vi "Add VI Reference Case.vi"(8 "error in":errorcluster, 11 "CSM-Helper in":refnum<class "CSM-Helper.lvclass">) -> (0 "error out":errorcluster, 3 "CSM-Helper out":refnum<class "CSM-Helper.lvclass">)   [LabVIEW 2017, in "CSM-Helper.lvclass"]
doc: "### Add VI Reference Case.vi\n\n-- <b>Controls</b> --\n- <b>CSM-Helper in</b>: CSMHelper input\n\n-- <b>Indicators</b> --\n- <b>CSM-Helper out</b>: CSMHelper output"
uses:
  CSM-Helper.lvclass
  API/Connect Paired Tunnels.vi
  API/Connect Error Wire If not Connected.vi
  API/Connect StateQ Wire If not Connected.vi
  API/Connect Internal Data Wire If not Connected.vi
  API/Connect EventReg Wire If not Connected.vi
  API/Add State Frame.vi
  API/Undo.vi
  API/Stop Undo.vi
  API/Start Undo.vi
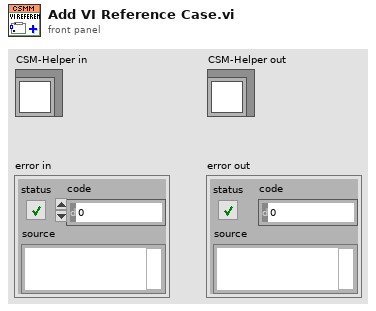
[diagram p1: front panel]
types:
  T1 = enum32{"Invalid", "Standard", "Closed", "Hidden", "Minimized", "Maximized"}
  T2 = enum32{"invalid app kind", "Development System", "Run Time System", "Student Edition", "Embedded LabVIEW", "Evaluation", "Custom"}
  T3 = cluster{"Core":cluster{"Current VI Reference":refnum<vi>, "Close Panel on Exit?":bool, "error":errorcluster}, "Frame":refnum<vi>}
  T4 = cluster{"Current VI Reference":refnum<vi>, "Close Panel on Exit?":bool, "error":errorcluster}
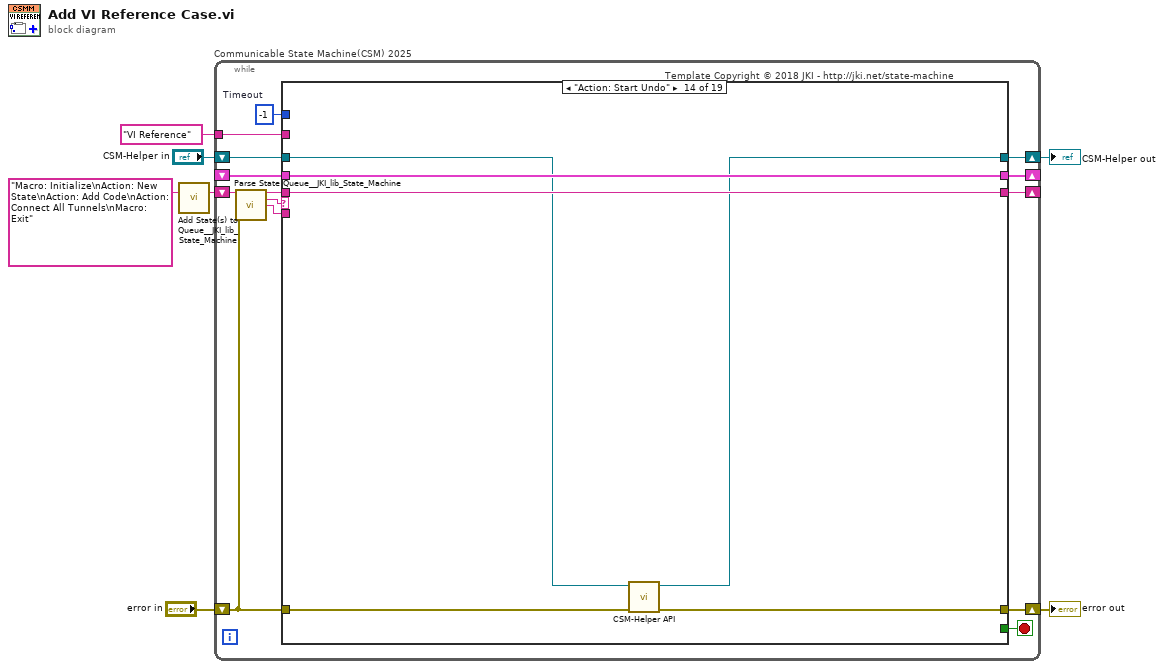
[diagram p0: block diagram]
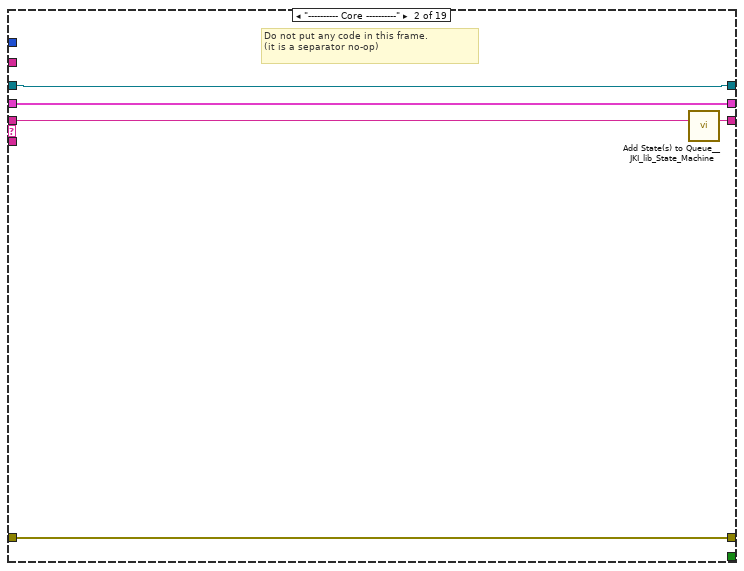
[diagram p3: hidden frame]
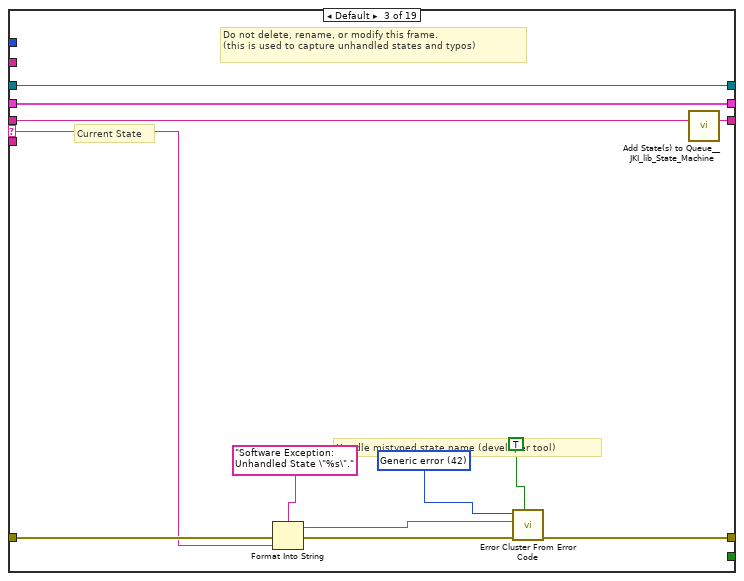
[diagram p4: hidden frame]
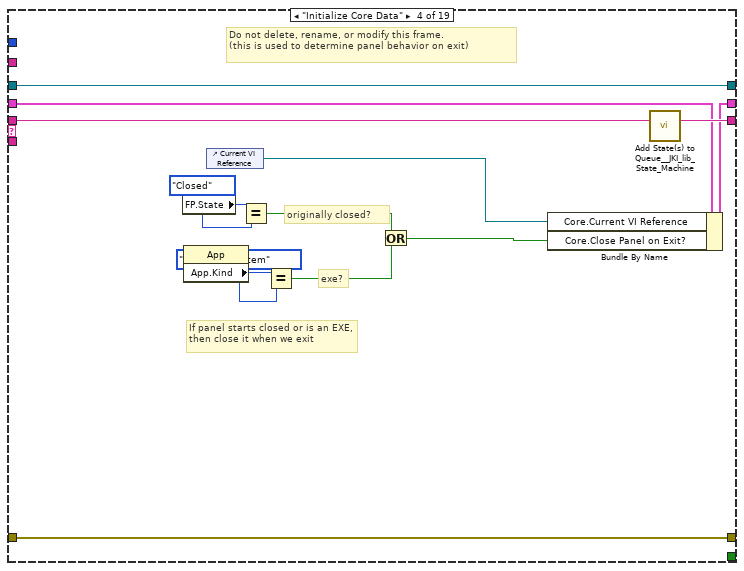
[diagram p5: hidden frame]
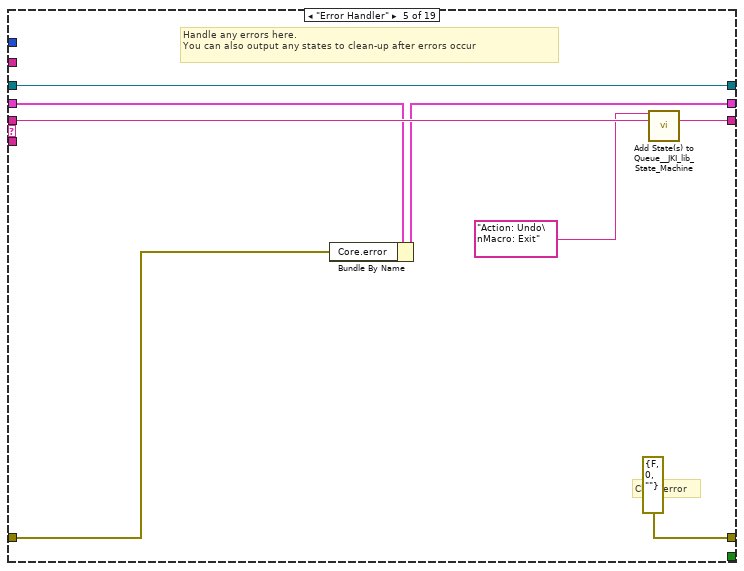
[diagram p6: hidden frame]
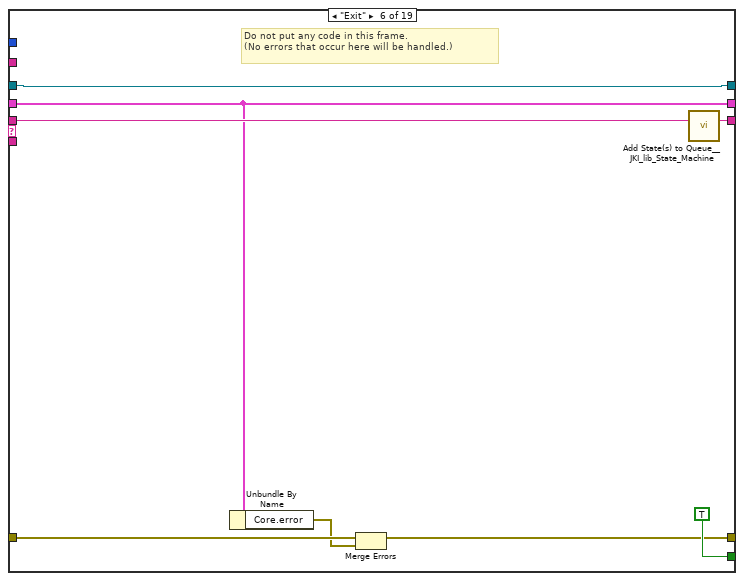
[diagram p7: hidden frame]
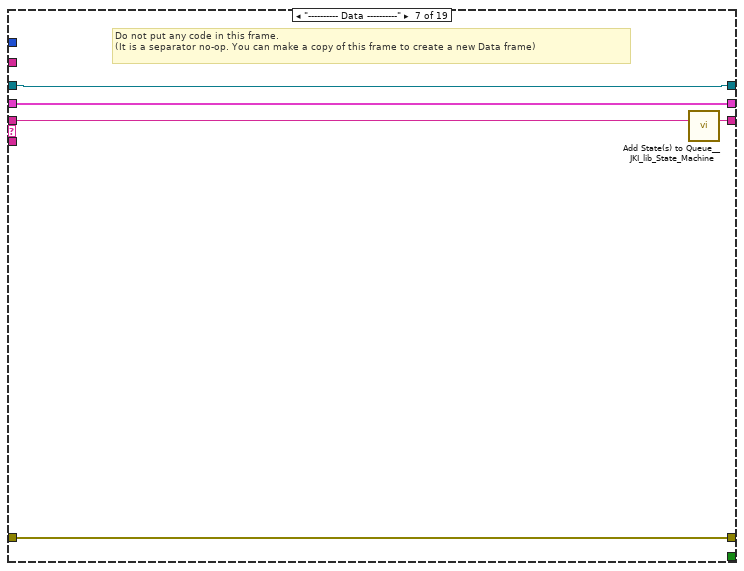
[diagram p8: hidden frame]
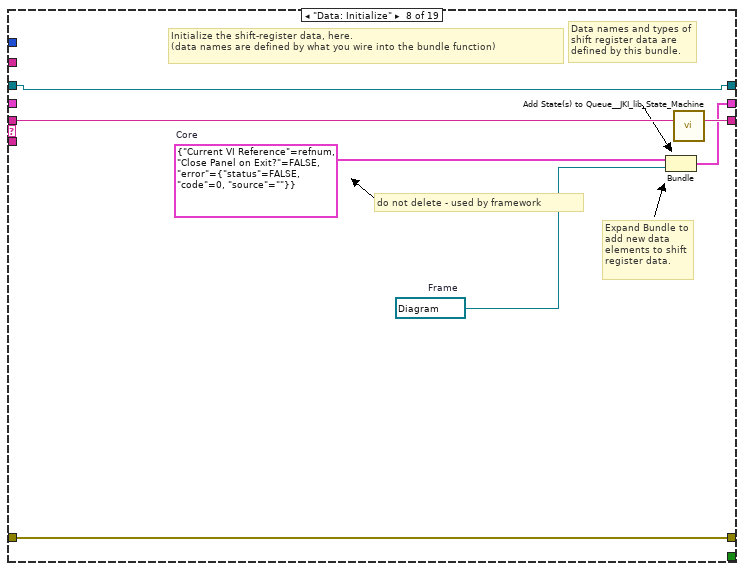
[diagram p9: hidden frame]
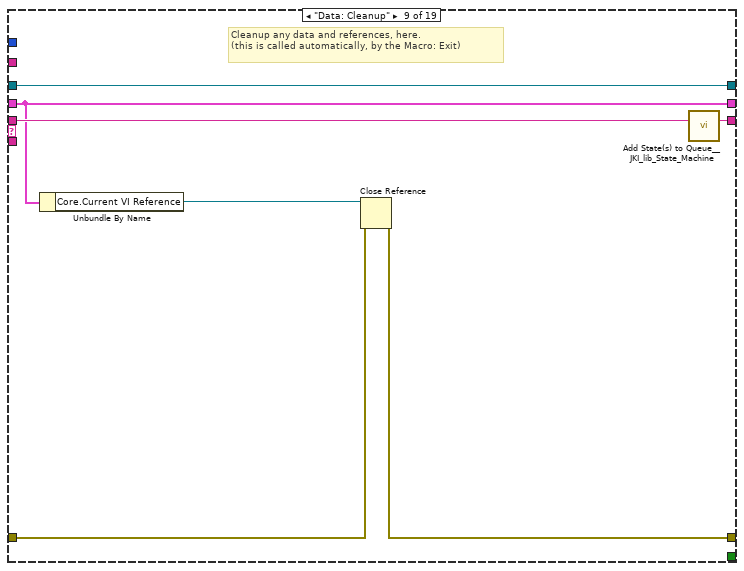
[diagram p10: hidden frame]
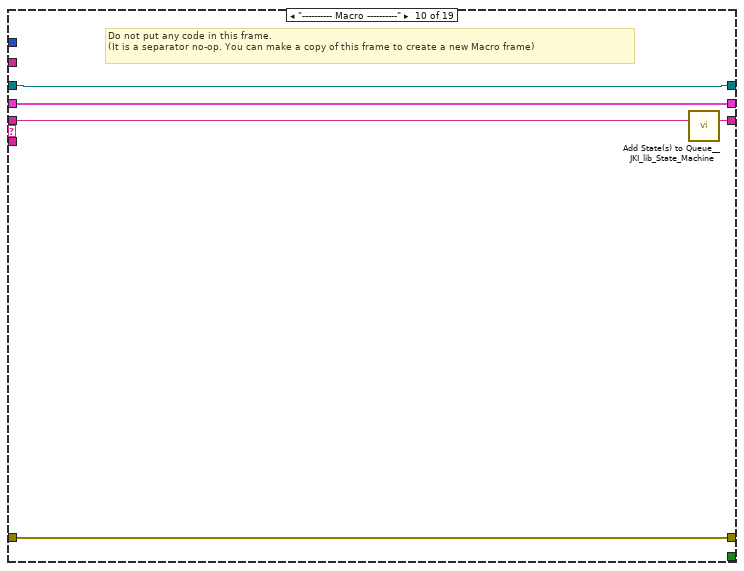
[diagram p11: hidden frame]
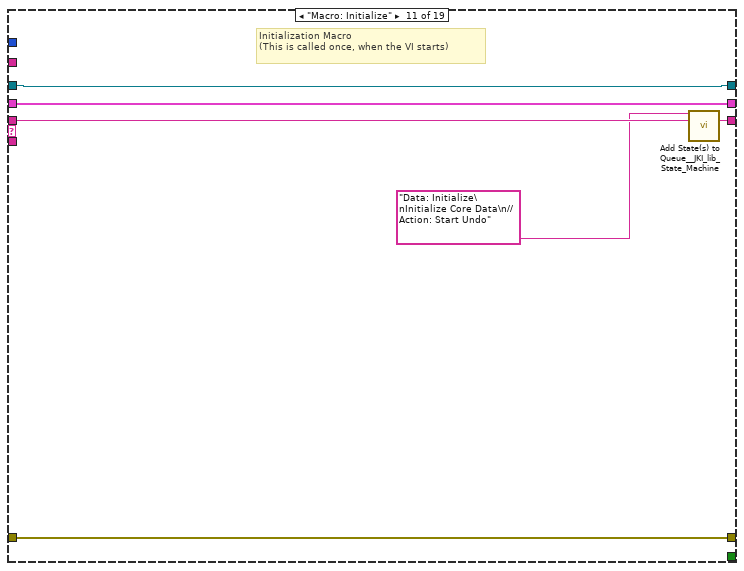
[diagram p12: hidden frame]
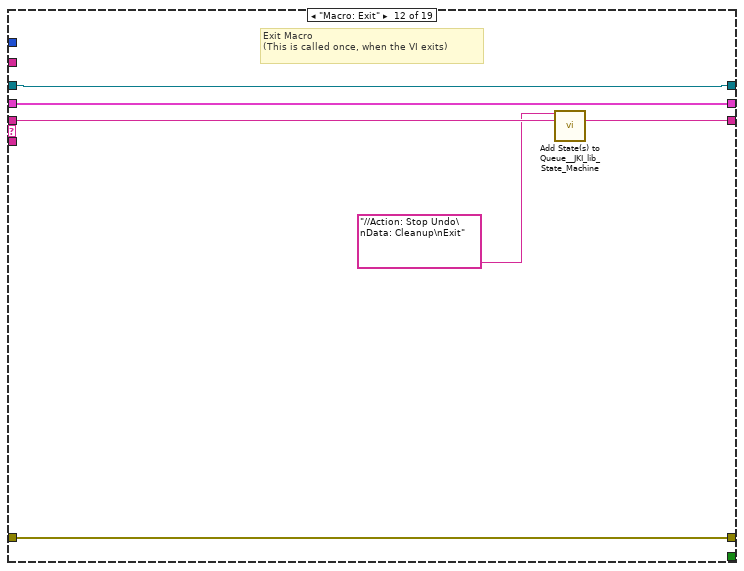
[diagram p13: hidden frame]
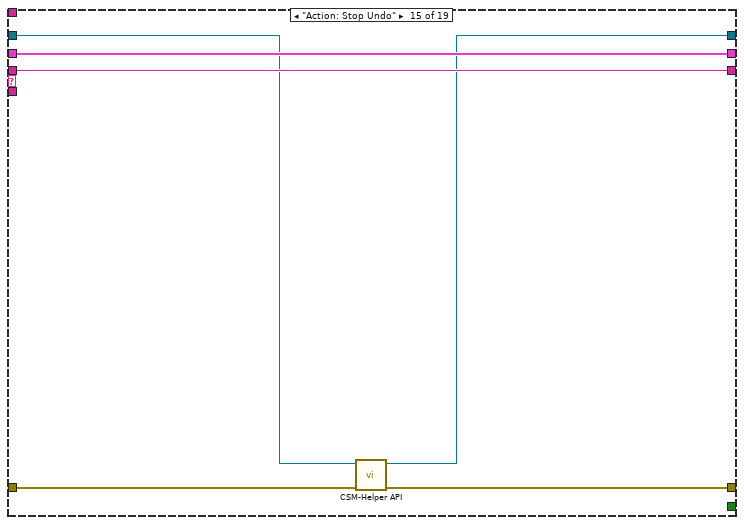
[diagram p15: hidden frame]
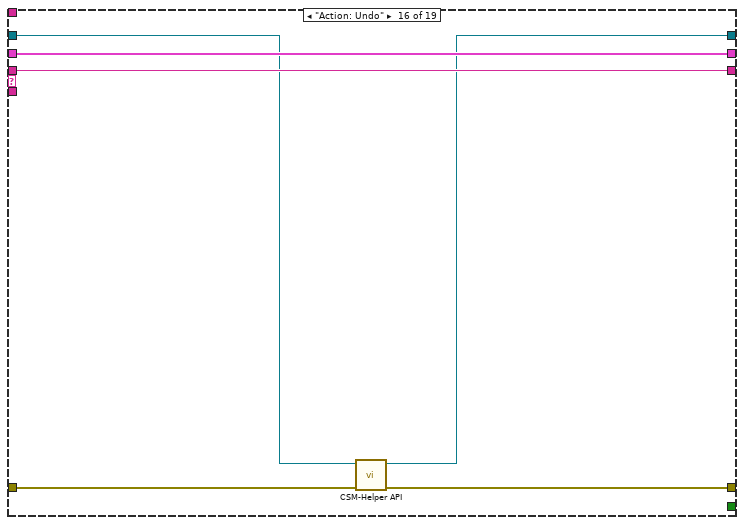
[diagram p16: hidden frame]
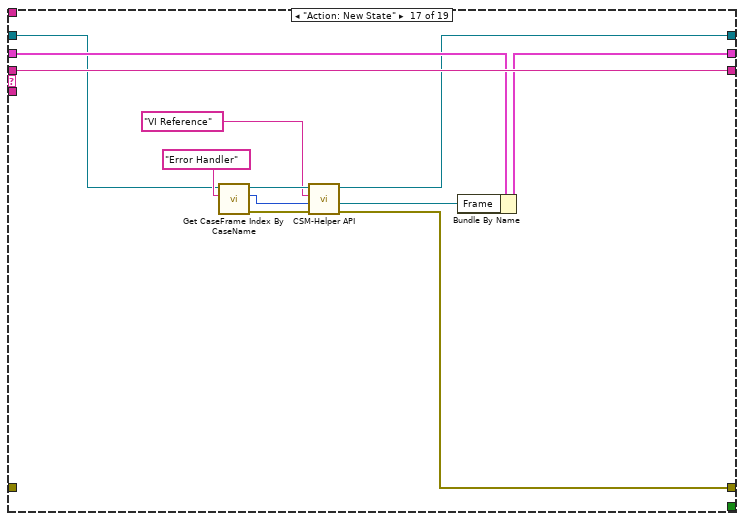
[diagram p17: hidden frame]
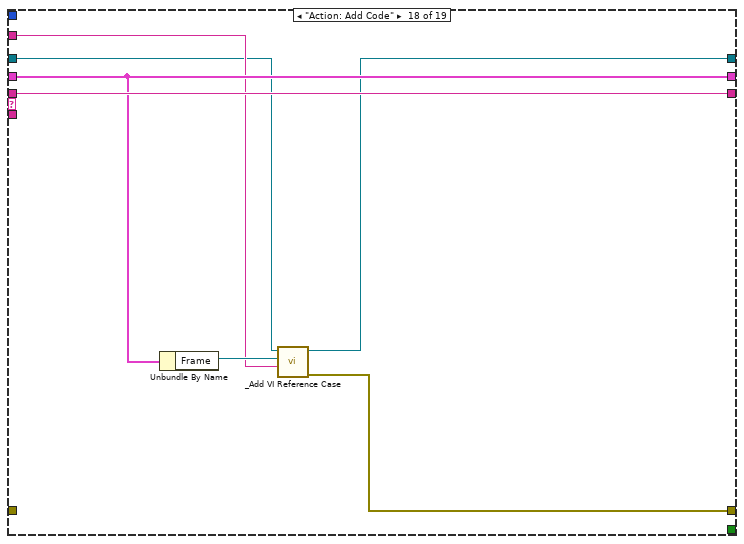
[diagram p18: hidden frame]
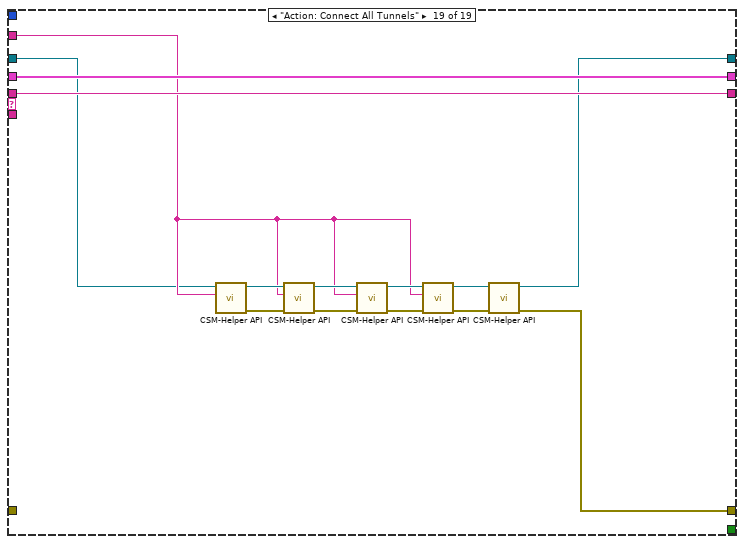
[diagram p19: hidden frame]
diagram:
  n1 = call <vilib>:"Add State(s) to Queue__JKI_lib_State_Machine.vi"("State(s) in (\"\")"="Macro: Initialize\nAction: New State\nAction: Add Code\nAction: Connect All Tunnels\nMacro: Exit") -> ("States Out"=w7:string)  [unwired: 14 in]
  n2 = while "Communicable State Machine(CSM) 2025" {
    shift-right: [w14] -> _
    shift-left: _ -> [w13]
    shift-right: [w17] -> w4
    shift-left: "error in" -> [w11]
    shift-right: [w16] -> _
    shift-left: w7 -> [w18]
    shift-right: [w9] -> w2
    shift-left: "CSM-Helper in" -> [w10]
    tunnel: "VI Reference" ("element") -> [w8]
    stop <- w15 stop-if-true
    w12 = -1  # Timeout
    # "Template Copyright © 2018 JKI - http://jki.net/state-machine"
    n3 = call <vilib>:"Parse State Queue__JKI_lib_State_Machine.vi"("State Queue"=w18, "Error In (no error)"=w11) -> ("Remaining States"=w20:string, "Current State"=w21:string, "Arguments"=w19:string)  [unwired: 11 in]
    n4 = case shown="\"Action: Start Undo\"" w21 {
      selector: w21 -> [_ _ w32 _ _ _ _ _ _ _ _ _ _ _ _ _ _ _ _]
      tunnel: w20 -> [w25 w30 w36 w56 w64 w72 w77 w84 w91 w96 w102 w108 w110 w117 w123 w129 w142 w149 w163]
      tunnel: w19 -> [_ _ _ _ _ _ _ _ _ _ _ _ _ _ _ _ _ _ _]
      tunnel: w13 -> [w23 w27 w34 w49 w61 w66 w74 _ w86 w93 w99 w105 w111 w118 w124 w130 w141 w148 w162]
      tunnel: [w24 w28 w38 w53 errorcluster {"status"=FALSE, "code"=0, "source"=""} ("error out") w67 w75 w81 w87 w94 w100 w106 w109 w115 w121 w127 w135 w143 w153] -> w17
      tunnel: w11 -> [w24 w28 w37 w53 w57 w70 w75 w81 w88 w94 w100 w106 w109 w116 w122 w128 _ _ _]
      tunnel: [w25 w29 w35 w55 w63 w71 w76 w83 w90 w95 w101 w107 w110 w117 w123 w129 w142 w149 w163] -> w16
      tunnel: [_ _ _ _ _ TRUE _ _ _ _ _ _ _ _ _ _ _ _ _] -> w15
      tunnel: [w23 w27 w34 w54 w58 w66 w74 w82 w86 w93 w99 w105 w111 w118 w124 w130 w132 w148 w162] -> w14
      tunnel: w12 -> [_ _ _ _ _ _ _ _ _ _ _ _ _ _ _ _ _ _ _]
      tunnel: w10 -> [w22 w26 w31 w43 w59 w68 w73 w79 w85 w92 w97 w103 w112 w114 w120 w126 w134 w145 w151]
      tunnel: [w22 w26 w31 w43 w59 w68 w73 w79 w85 w92 w97 w103 w112 w113 w119 w125 w133 w144 w150] -> w9
      tunnel: w8 -> [_ _ _ _ _ _ _ _ _ _ _ _ _ _ _ _ _ w146 w152]
      frame "", "Event Structure", "Idle" {
        # "executes when the state queue is empty"
      }
      frame "---------- Core ----------" {
        # "Do not put any code in this frame.\n(it is a separator no-op)"
        n5 = call <vilib>:"Add State(s) to Queue__JKI_lib_State_Machine.vi"("State(s) in (\"\")"=w30) -> ("States Out"=w29:string)  [unwired: 14 in]
      }
      frame Default {
        w41 = 42 items=["No error", "Argument error", "Memory is full", "Out of zone", "End of file", "File already open", "Generic file I/O error", "File not found", "File permission error", "Disk is full", "Duplicate path", "Too many files open", "System feature not enabled", "Resource file not found", "Cannot add resource", "Resource not found", "Image not found", "Image memory error", "Pen does not exist", "Config type invalid", "Config token not found", "Config parse error", "Config memory error", "Bad external code format", "Bad external code offset", "External code not present", "Null window", "Destroy window error", "Null menu", "Print aborted", "Bad print record", "Print driver error", "Windows error during printing", "Memory error during printing", "Print dialog error", "Generic print error", "Invalid device refnum", "Device not found", "Device parameter error", "Device unit error", "Cannot open device", "Device call aborted", "Generic error", "Cancelled by user", "Object ID too low", "Object ID too high", "Object not in heap", "Unknown heap", "Unknown object (invalid DefProc)", "Unknown object (DefProc not in table)", "Message out of range", "Invalid (null) method", "Unknown message", "Manager call not supported", "Bad address", "Network operation in progress", "Network operation timed out", "Connection is busy", "Network attribute not supported", "Network error", "Address in use", "System out of memory", "Connection aborted", "Connection refused", "Not connected", "Already connected", "Connection closed", "Initialization error (interapplication manager)", "Bad occurrence", "Wait on unbound occurrence handler", "Occurrence queue overflow", "Datalog type conflict", "Unused", "Unrecognized type (interapplication manager)", "Memory corrupt", "Failed to make temporary DLL", "Old CIN version", "Drag socket not found", "Failed to load drop-object", "Failed to register OLE object", "Failed to release OLE object", "Format specifier type mismatch", "Unknown format specifier", "Too few format specifiers", "Too many format specifiers", "Scan failed", "Newer CIN version", "Error converting to variant", "Runtime menu error", "Password tampered", "Variant attribute not found", "Incompatible variant data type", "Event data is not available", "Event Store is not present", "Occurrence is not found", "Event Queue is not created", "Event info is not available", "Refnum passed is NULL", "Error retrieving Class GUID", "Error retrieving CoClass GUID", "Error retrieving TypeLib GUID.", "Bad built application magic bytes.", "Specific driver is different from the specific driver associated with the Logical Name.", "There is no session opened to the class driver.", "Max Error", "MAX - Error with config objects", "MAX - Error loading configuration", "MAX - Group not supported"]
        # "Current State"
        # "Do not delete, rename, or modify this frame.\n(this is used to capture unhandled states and typos)"
        # "Handle mistyped state name (developer tool)"
        n6 = Format Into String(format string="Software Exception: Unhandled State \"%s\"." ("message"), error in=w37, w32) -> (resulting string=w40:string, error out=w39:errorcluster)  [unwired: 1 in]
        n7 = call <vilib>:"Error Cluster From Error Code.vi"("show call chain? (False)"=TRUE, "error in (no error)"=w39, "error message (\"\")"=w40, "error code (0)"=w41) -> ("error out"=w38:errorcluster)  [unwired: 5 in]
        n8 = call <vilib>:"Add State(s) to Queue__JKI_lib_State_Machine.vi"("State(s) in (\"\")"=w36) -> ("States Out"=w35:string)  [unwired: 14 in]
      }
      frame "Initialize Core Data" {
        # "Do not delete, rename, or modify this frame.\n(this is used to determine panel behavior on exit)"
        # "originally closed?"
        # "exe?"
        # "If panel starts closed or is an EXE, then close it when we exit"
        n9 = property class="VI"() -> ("FP.State"=w46:T1)  [unwired: 2 in, 2 out]
        n10 = property class="App"() -> ("App.Kind"=w52:T2)  [unwired: 2 in, 2 out]
        n11 = control-ref of="Current VI Reference"() -> (w47:refnum<vi>)
        n12 = Equal?(x=w46, y=T1."Closed" ("Front Panel Window:State")) -> (x = y?=w44:bool)
        n13 = Equal?(x=w52, y=T2."Run Time System" ("Application:Kind")) -> (x = y?=w50:bool)
        n14 = Or(x=w44, y=w50) -> (x .or. y?=w48:bool)
        n15 = Bundle By Name(cluster=w49, "Core.Current VI Reference"=w47, "Core.Close Panel on Exit?"=w48) -> (w54:T3)
        n16 = call <vilib>:"Add State(s) to Queue__JKI_lib_State_Machine.vi"("State(s) in (\"\")"=w56) -> ("States Out"=w55:string)  [unwired: 14 in]
      }
      frame "Error Handler" {
        # "Handle any errors here.\nYou can also output any states to clean-up after errors occur"
        # "Clear error"
        n17 = Bundle By Name(cluster=w61, "Core.error"=w57) -> (w58:T3)
        n18 = call <vilib>:"Add State(s) to Queue__JKI_lib_State_Machine.vi"("State(s) in Front (\"\")"="Action: Undo\nMacro: Exit", "State(s) in (\"\")"=w64) -> ("States Out"=w63:string)  [unwired: 13 in]
      }
      frame "Exit" {
        # "Do not put any code in this frame.\n(No errors that occur here will be handled.)"
        n19 = Unbundle By Name(w66) -> ("Core.error"=w65:errorcluster)
        n20 = Merge Errors(w70, w65) -> (w67:errorcluster)
        n21 = call <vilib>:"Add State(s) to Queue__JKI_lib_State_Machine.vi"("State(s) in (\"\")"=w72) -> ("States Out"=w71:string)  [unwired: 14 in]
      }
      frame "---------- Data ----------" {
        # "Do not put any code in this frame.\n(It is a separator no-op. You can make a copy of this frame to create a new Data frame)"
        n22 = call <vilib>:"Add State(s) to Queue__JKI_lib_State_Machine.vi"("State(s) in (\"\")"=w77) -> ("States Out"=w76:string)  [unwired: 14 in]
      }
      frame "Data: Initialize" {
        w78 = refnum<vi> refnum  # Frame
        w80 = T4 {"Current VI Reference"=refnum, "Close Panel on Exit?"=FALSE, "error"={"status"=FALSE, "code"=0, "source"=""}}  # Core
        # "do not delete - used by framework"
        # "Expand Bundle to add new data elements to shift register data."
        # "Data names and types of shift register data are defined by this bundle."
        # "Initialize the shift-register data, here.\n(data names are defined by what you wire into the bundle function)"
        n23 = Bundle("Core"=w80, "Frame"=w78) -> (w82:T3)  [unwired: 1 in]
        n24 = call <vilib>:"Add State(s) to Queue__JKI_lib_State_Machine.vi"("State(s) in (\"\")"=w84) -> ("States Out"=w83:string)  [unwired: 14 in]
      }
      frame "Data: Cleanup" {
        # "Cleanup any data and references, here.\n(this is called automatically, by the Macro: Exit)"
        n25 = Unbundle By Name(w86) -> ("Core.Current VI Reference"=w89:refnum<vi>)
        n26 = Close Reference(reference=w89, error in (no error)=w88) -> (error out=w87:errorcluster)
        n27 = call <vilib>:"Add State(s) to Queue__JKI_lib_State_Machine.vi"("State(s) in (\"\")"=w91) -> ("States Out"=w90:string)  [unwired: 14 in]
      }
      frame "---------- Macro ----------" {
        # "Do not put any code in this frame.\n(It is a separator no-op. You can make a copy of this frame to create a new Macro frame)"
        n28 = call <vilib>:"Add State(s) to Queue__JKI_lib_State_Machine.vi"("State(s) in (\"\")"=w96) -> ("States Out"=w95:string)  [unwired: 14 in]
      }
      frame "Macro: Initialize" {
        # "Initialization Macro\n(This is called once, when the VI starts)"
        n29 = call <vilib>:"Add State(s) to Queue__JKI_lib_State_Machine.vi"("State(s) in Front (\"\")"="Data: Initialize\nInitialize Core Data\n//Action: Start Undo", "State(s) in (\"\")"=w102) -> ("States Out"=w101:string)  [unwired: 13 in]
      }
      frame "Macro: Exit" {
        # "Exit Macro\n(This is called once, when the VI exits)"
        n30 = call <vilib>:"Add State(s) to Queue__JKI_lib_State_Machine.vi"("State(s) in Front (\"\")"="//Action: Stop Undo\nData: Cleanup\nExit", "State(s) in (\"\")"=w108) -> ("States Out"=w107:string)  [unwired: 13 in]
      }
      frame "--------- Action -----------" {
      }
      frame "Action: Start Undo" {
        n31 = call-poly "CSM-Helper API.vi"("error in (no error)"=w116, "CSM-Helper in"=w114) -> ("error out"=w115:errorcluster, "CSM-Helper out"=w113:refnum<class "CSM-Helper.lvclass">)  [unwired: 8 in]
      }
      frame "Action: Stop Undo" {
        n32 = call-poly "CSM-Helper API.vi"("error in (no error)"=w122, "CSM-Helper in"=w120) -> ("error out"=w121:errorcluster, "CSM-Helper out"=w119:refnum<class "CSM-Helper.lvclass">)  [unwired: 8 in]
      }
      frame "Action: Undo" {
        n33 = call-poly "CSM-Helper API.vi"("error in (no error)"=w128, "CSM-Helper in"=w126) -> ("error out"=w127:errorcluster, "CSM-Helper out"=w125:refnum<class "CSM-Helper.lvclass">)  [unwired: 8 in]
      }
      frame "Action: New State" {
        n34 = call "Get CaseFrame Index By CaseName.vi"("CASE"="Error Handler" ("Frame Name"), "CSM-Helper in"=w134) -> ("error out"=w137:errorcluster, "index"=w140:i32, "CSM-Helper out"=w138:refnum<class "CSM-Helper.lvclass">)  [unwired: 6 in, 1 out]
        n35 = call-poly "CSM-Helper API.vi"("error in (no error)"=w137, "index(-1, use same group)"=w140, "element"="VI Reference", "CSM-Helper in"=w138) -> ("error out"=w135:errorcluster, "Add Frame"=w131:refnum<vi>, "CSM-Helper out"=w133:refnum<class "CSM-Helper.lvclass">)  [unwired: 5 in]
        n36 = Bundle By Name(cluster=w141, "Frame"=w131) -> (w132:T3)
      }
      frame "Action: Add Code" {
        n37 = Unbundle By Name(w148) -> ("Frame"=w147:refnum<vi>)
        n38 = call "_Add VI Reference Case.vi"("element"=w146, "Add Frame"=w147, "CSM-Helper in"=w145) -> ("error out"=w143:errorcluster, "CSM-Helper out"=w144:refnum<class "CSM-Helper.lvclass">)  [unwired: 7 in]
      }
      frame "Action: Connect All Tunnels" {
        n39 = call-poly "CSM-Helper API.vi"("case"=w152, "CSM-Helper in"=w151) -> ("error out"=w159:errorcluster, "CSM-Helper out"=w158:refnum<class "CSM-Helper.lvclass">)  [unwired: 8 in]
        n40 = call-poly "CSM-Helper API.vi"("error in (no error)"=w159, "case"=w152, "CSM-Helper in"=w158) -> ("error out"=w156:errorcluster, "CSM-Helper out"=w157:refnum<class "CSM-Helper.lvclass">)  [unwired: 7 in]
        n41 = call-poly "CSM-Helper API.vi"("error in (no error)"=w156, "case"=w152, "CSM-Helper in"=w157) -> ("error out"=w154:errorcluster, "CSM-Helper out"=w155:refnum<class "CSM-Helper.lvclass">)  [unwired: 7 in]
        n42 = call-poly "CSM-Helper API.vi"("error in (no error)"=w154, "case"=w152, "CSM-Helper in"=w155) -> ("error out"=w160:errorcluster, "CSM-Helper out"=w161:refnum<class "CSM-Helper.lvclass">)  [unwired: 7 in]
        n43 = call-poly "CSM-Helper API.vi"("error in (no error)"=w160, "CSM-Helper in"=w161) -> ("error out"=w153:errorcluster, "CSM-Helper out"=w150:refnum<class "CSM-Helper.lvclass">)  [unwired: 8 in]
      }
    }
  }
  "error out" <- w4
  "CSM-Helper out" <- w2
